vi "Read Parameters to process.vi"(8 "error in":errorcluster, 11 "My Awesome Control Modules runtime in":refnum<class "My Awesome Control Modules runtime.lvclass">) -> (0 "error out":errorcluster, 2 "Parameters to process":T1, 3 "My Awesome Control Modules runtime out":refnum<class "My Awesome Control Modules runtime.lvclass">)   [LabVIEW 2013, in "My Awesome Control Modules runtime.lvclass"]
uses:
  My Awesome Control Modules runtime.lvclass
  configuration/parameter data indices.ctl
  configuration/My Awesome Control Modules configuration.lvclass
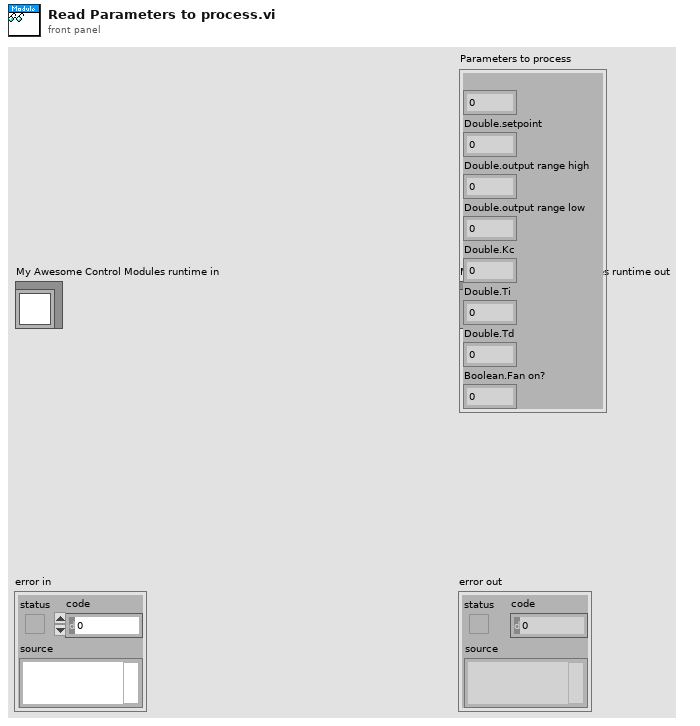
[diagram p1: front panel]
types:
  T1 = typedef "My Awesome Control Modules configuration.lvclass/parameter data indices.ctl" = cluster{"Double.Temperature":i32, "Double.setpoint":i32, "Double.output range high":i32, "Double.output range low":i32, "Double.Kc":i32, "Double.Ti":i32, "Double.Td":i32, "Boolean.Fan on?":i32}
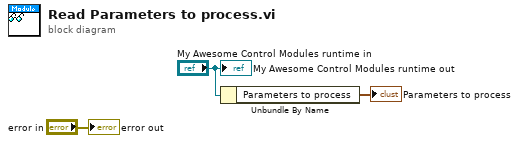
[diagram p0: block diagram]
diagram:
  n1 = Unbundle By Name("My Awesome Control Modules runtime in") -> ("Parameters to process"=→"Parameters to process":T1)
  "error out" <- "error in"
  "My Awesome Control Modules runtime out" <- "My Awesome Control Modules runtime in"
